vi "Get Copyright Path.vi"(8 "error in (no error)":errorcluster) -> (0 "error out":errorcluster, 3 "Copyright Path":path)   [LabVIEW 2023, in "VI Properties Editor.lvlib"]
doc: "Gets copyright path."
uses:
  <vilib>/Utility/sysdir.llb/System Directory Type.ctl
  VI Properties Editor.lvlib
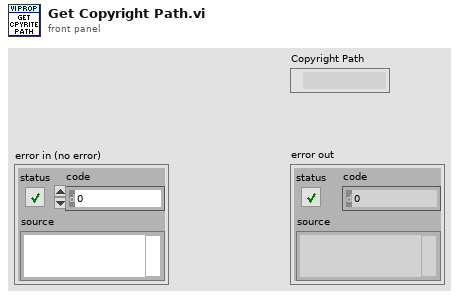
[diagram p1: front panel]
types:
  T1 = typedef "System Directory Type.ctl" = i32
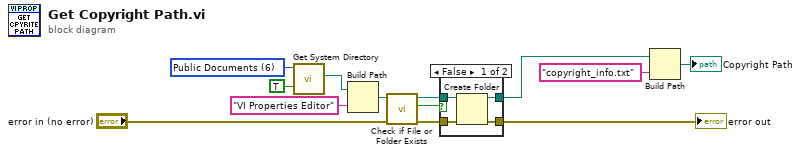
[diagram p0: block diagram]
diagram:
  w1 = T1 6 items=["User Home"=0, "User Desktop"=1, "User Documents"=2, "User Application Data"=3, "User Preferences"=4, "User Temporary"=5, "Public Documents"=6, "Public Application Data"=7, "Public Preferences"=8, "Public Cache"=13, "System Core Libraries"=9, "System Installed Libraries"=10, "Application Files"=11, "Boot Volume Root"=12] ("system directory type")
  n1 = call <vilib>:"Get System Directory.vi"("create directory if not found? (F)"=TRUE, "system directory type"=w1) -> ("system directory"=w3:path)  [unwired: 9 in]
  n2 = Build Path(base path=w3, name or relative path="VI Properties Editor") -> (appended path=w6:path)
  n3 = call <vilib>:"Check if File or Folder Exists.vi"("error in (no error)"="error in (no error)", "path"=w6) -> ("error out"=w9:errorcluster, "file or folder exists?"=w7:bool, "dup path"=w8:path)  [unwired: 7 in]
  n4 = case shown="False" w7 {
    tunnel: w8 -> [w17 w19]
    tunnel: w9 -> [w16 w18]
    tunnel: [w15 w18] -> w13
    tunnel: [w14 w19] -> w10
    frame False {
      n5 = Create Folder(path (use dialog)=w17, error in=w16) -> (created path=w14:path, error out=w15:errorcluster)  [unwired: 1 in, 1 out]
    }
    frame True {
    }
  }
  "error out" <- w13
  n6 = Build Path(base path=w10, name or relative path="copyright_info.txt") -> (appended path=→"Copyright Path":path)
